vi "Initial AI Voltage.vi"(8 "error in":errorcluster, 11 "AI Properties":T1 {"AI Signals properties Array"."Input Configuration" items=["RSE"=10083, "NRSE"=10078, "Differential"=10106]}) -> (0 "error out":errorcluster, 3 "DAQ Ref out":refnum<k21>)   [LabVIEW 2021, in "DAQ Analog InOut Engine.lvlib"]
uses:
  DAQ Analog InOut Engine.lvlib
  AI Properties.ctl
  System Explorer/Types/Input Channel Parameters.ctl
  <vilib>/DAQmx/create/channels.llb/DAQmx Create Channel (AI-Voltage-Basic).vi
  <resource>/objmgr/daqmx.rc
  System Explorer/DAQ Analog InOut System Explorer.lvlib
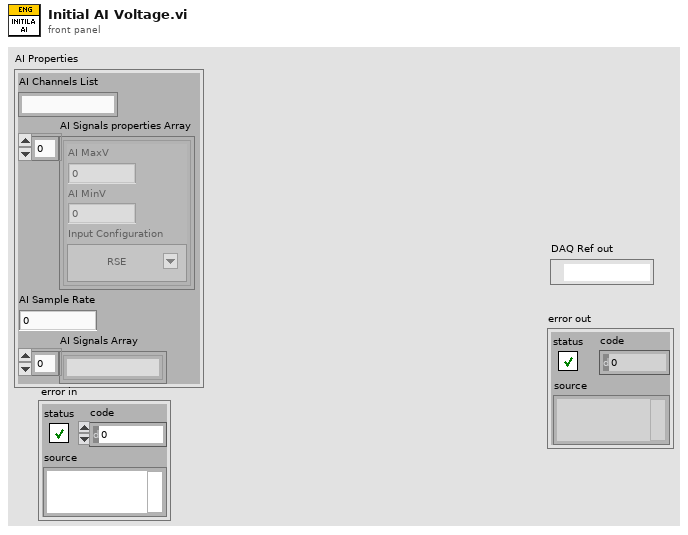
[diagram p1: front panel]
types:
  T1 = typedef "DAQ Analog InOut Engine.lvlib/AI Properties.ctl" = cluster{"AI Channels List":string, "AI Signals properties Array":T2[], "AI Sample Rate":dbl, "AI Signals Array":string[]}
  T2 = typedef "DAQ Analog InOut System Explorer.lvlib/Input Channel Parameters.ctl" = cluster{"AI MaxV":dbl, "AI MinV":dbl, "Input Configuration":u16}
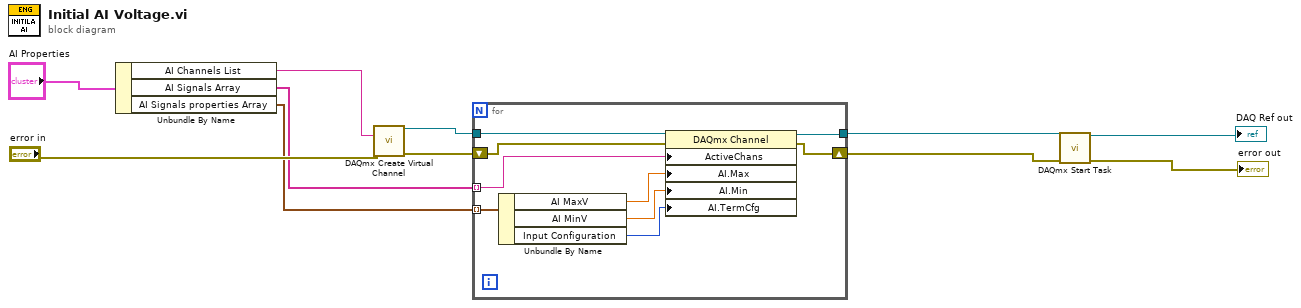
[diagram p0: block diagram]
diagram:
  n1 = Unbundle By Name("AI Properties") -> ("AI Channels List"=w3:string, "AI Signals Array"=w4:string[], "AI Signals properties Array"=w5:T2[])
  n2 = call-poly <vilib>:"DAQmx Create Virtual Channel.vi"("physical channels"=w3, "error in"="error in") -> ("task out"=w7:refnum<k21>, "error out"=w6:errorcluster)  [unwired: 12 in]
  n3 = for {
    shift-right: [w18] -> w1
    shift-left: w6 -> [w19]
    tunnel: w4 -> [w16] mode=indexing
    tunnel: w5 -> [w15] mode=indexing
    tunnel: w7 -> [w20]
    tunnel: [w17] -> w2
    n4 = Unbundle By Name(w15) -> ("AI MaxV"=w14:dbl, "AI MinV"=w13:dbl, "Input Configuration"=w12:u16)
    n5 = property class="DAQmx Channel"(reference=w20, error in=w19, "ActiveChans"=w16, "AI.Max"=w14, "AI.Min"=w13, "AI.TermCfg"=w12) -> (reference out=w17:refnum<k21>, error out=w18:errorcluster)
  }
  n6 = call <vilib>:"DAQmx Start Task.vi"("task/channels in"=w2, "error in"=w1) -> ("task out"=→"DAQ Ref out":refnum<k21>, "error out"=→"error out":errorcluster)  [unwired: 12 in]
